vi "LED 7segment Example 1.vi"() -> ()   [LabVIEW 2014]
doc: "Light up 7segment LED."
panel:
  out "error out":errorcluster
  in  "error in":errorcluster
  # "+----------+\n|                |\n|                |\n|                |\n+----------+\n|                |\n|                |\n|                |\n+----------+ +"
  # "pin 9"
  # "pin 8"
  # "pin 10"
  # "pin 7"
  # "pin 6"
  # "pin 3"
  # "pin 4"
  # "pin 2"
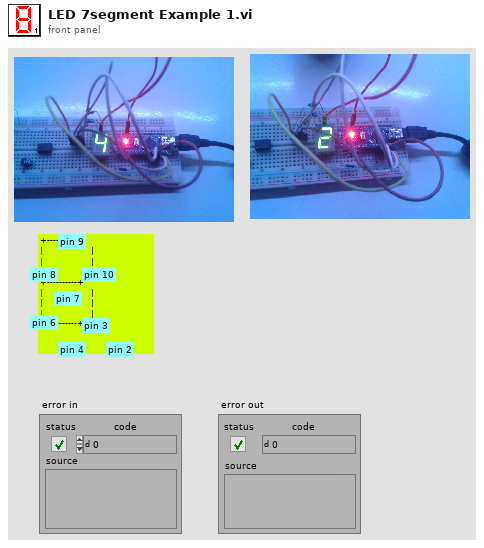
[diagram p1: front panel]
types:
  T1 = enum16{"nothing", "0", "1", "2", "3", "4", "5", "6", "7", "8", "9", "A", "B", "C", "D", "E", "F", "J", "L", "O", "P", "S", "U"}
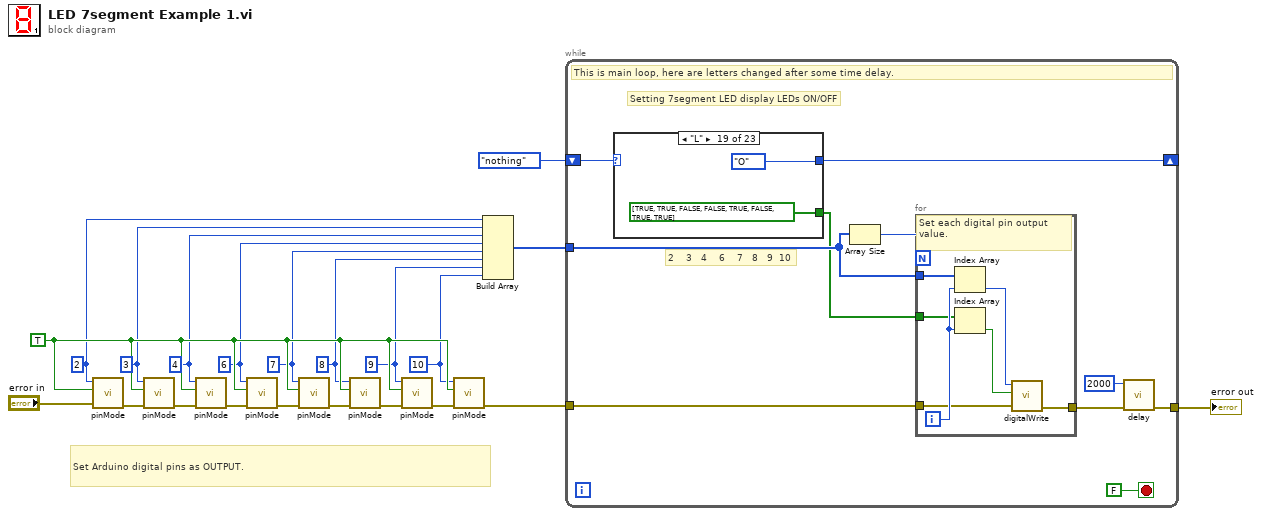
[diagram p0: block diagram]
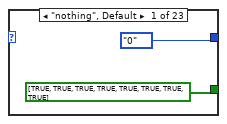
[diagram p2: hidden frame]
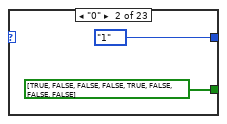
[diagram p3: hidden frame]
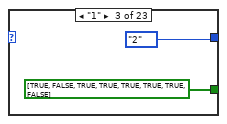
[diagram p4: hidden frame]
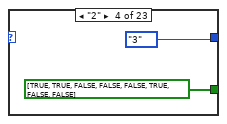
[diagram p5: hidden frame]
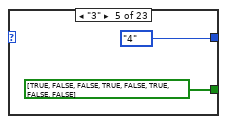
[diagram p6: hidden frame]
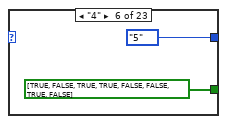
[diagram p7: hidden frame]
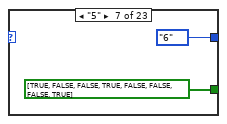
[diagram p8: hidden frame]
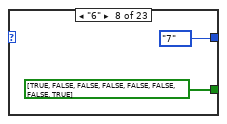
[diagram p9: hidden frame]
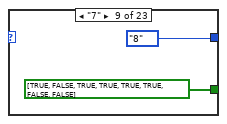
[diagram p10: hidden frame]
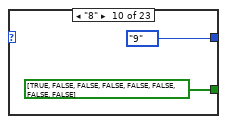
[diagram p11: hidden frame]
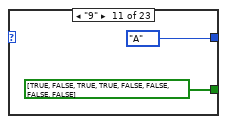
[diagram p12: hidden frame]
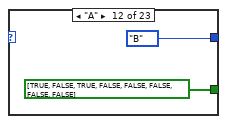
[diagram p13: hidden frame]
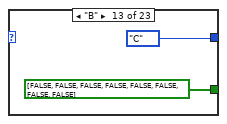
[diagram p14: hidden frame]
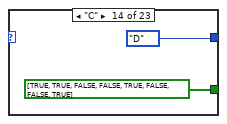
[diagram p15: hidden frame]
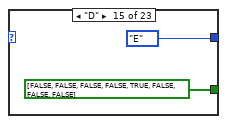
[diagram p16: hidden frame]
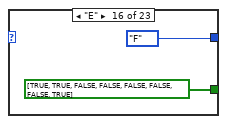
[diagram p17: hidden frame]
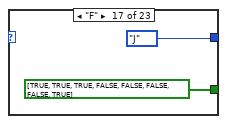
[diagram p18: hidden frame]
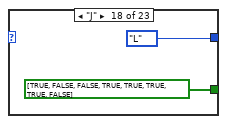
[diagram p19: hidden frame]
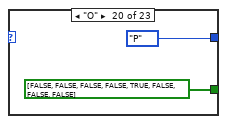
[diagram p20: hidden frame]
diagram:
  w3 = 10 ("pin number")
  w4 = 9 ("pin number")
  w5 = 8 ("pin number")
  w6 = 7 ("pin number")
  w7 = 6 ("pin number")
  w8 = 4 ("pin number")
  w9 = 3 ("pin number")
  w10 = 2 ("pin number")
  w13 = TRUE ("output?")
  # "Set Arduino digital pins as OUTPUT."
  n1 = call <vilib>:"pinMode.vi"("Error In"="error in", "output?"=w13, "pin number"=w10) -> ("Error Out"=w20:errorcluster)  [unwired: 8 in]
  n2 = call <vilib>:"pinMode.vi"("Error In"=w20, "output?"=w13, "pin number"=w9) -> ("Error Out"=w14:errorcluster)  [unwired: 8 in]
  n3 = call <vilib>:"pinMode.vi"("Error In"=w14, "output?"=w13, "pin number"=w8) -> ("Error Out"=w19:errorcluster)  [unwired: 8 in]
  n4 = call <vilib>:"pinMode.vi"("Error In"=w19, "output?"=w13, "pin number"=w7) -> ("Error Out"=w18:errorcluster)  [unwired: 8 in]
  n5 = call <vilib>:"pinMode.vi"("Error In"=w18, "output?"=w13, "pin number"=w6) -> ("Error Out"=w16:errorcluster)  [unwired: 8 in]
  n6 = call <vilib>:"pinMode.vi"("Error In"=w16, "output?"=w13, "pin number"=w5) -> ("Error Out"=w15:errorcluster)  [unwired: 8 in]
  n7 = call <vilib>:"pinMode.vi"("Error In"=w15, "output?"=w13, "pin number"=w4) -> ("Error Out"=w17:errorcluster)  [unwired: 8 in]
  n8 = call <vilib>:"pinMode.vi"("Error In"=w17, "output?"=w13, "pin number"=w3) -> ("Error Out"=w11:errorcluster)  [unwired: 8 in]
  n9 = Build Array(w10, w9, w8, w7, w6, w5, w4, w3) -> (w2:i32[])
  n10 = while {
    tunnel: [w30] -> w21
    tunnel: w11 -> [w27]
    tunnel: w2 -> [w28]
    shift-right: [w23] -> _
    shift-left: T1."nothing" -> [w24]
    stop <- FALSE stop-if-true
    # "Setting 7segment LED display LEDs ON/OFF"
    # "2    3   4    6    7   8   9  10"
    # "This is main loop, here are letters changed after some time delay."
    n11 = case shown="\"L\"" w24 {
      tunnel: [T1."0" T1."1" T1."2" T1."3" T1."4" T1."5" T1."6" T1."7" T1."8" T1."9" T1."A" T1."B" T1."C" T1."D" T1."E" T1."F" T1."J" T1."L" T1."O" T1."P" T1."S" T1."U" T1."nothing"] -> w23
      tunnel: [bool[] [TRUE, TRUE, TRUE, TRUE, TRUE, TRUE, TRUE, TRUE] bool[] [TRUE, FALSE, FALSE, FALSE, TRUE, FALSE, FALSE, FALSE] bool[] [TRUE, FALSE, TRUE, TRUE, TRUE, TRUE, TRUE, FALSE] bool[] [TRUE, TRUE, FALSE, FALSE, FALSE, TRUE, FALSE, FALSE] bool[] [TRUE, FALSE, FALSE, TRUE, FALSE, TRUE, FALSE, FALSE] bool[] [TRUE, FALSE, TRUE, TRUE, FALSE, FALSE, TRUE, FALSE] bool[] [TRUE, FALSE, FALSE, TRUE, FALSE, FALSE, FALSE, TRUE] bool[] [TRUE, FALSE, FALSE, FALSE, FALSE, FALSE, FALSE, TRUE] bool[] [TRUE, FALSE, TRUE, TRUE, TRUE, TRUE, FALSE, FALSE] bool[] [TRUE, FALSE, FALSE, FALSE, FALSE, FALSE, FALSE, FALSE] bool[] [TRUE, FALSE, TRUE, TRUE, FALSE, FALSE, FALSE, FALSE] bool[] [TRUE, FALSE, TRUE, FALSE, FALSE, FALSE, FALSE, FALSE] bool[] [FALSE, FALSE, FALSE, FALSE, FALSE, FALSE, FALSE, FALSE] bool[] [TRUE, TRUE, FALSE, FALSE, TRUE, FALSE, FALSE, TRUE] bool[] [FALSE, FALSE, FALSE, FALSE, TRUE, FALSE, FALSE, FALSE] bool[] [TRUE, TRUE, FALSE, FALSE, FALSE, FALSE, FALSE, TRUE] bool[] [TRUE, TRUE, TRUE, FALSE, FALSE, FALSE, FALSE, TRUE] bool[] [TRUE, FALSE, FALSE, TRUE, TRUE, TRUE, TRUE, FALSE] bool[] [TRUE, TRUE, FALSE, FALSE, TRUE, FALSE, TRUE, TRUE] bool[] [FALSE, FALSE, FALSE, FALSE, TRUE, FALSE, FALSE, FALSE] bool[] [TRUE, TRUE, TRUE, FALSE, FALSE, FALSE, FALSE, FALSE] bool[] [TRUE, FALSE, FALSE, TRUE, FALSE, FALSE, FALSE, TRUE] bool[] [TRUE, FALSE, FALSE, FALSE, TRUE, FALSE, TRUE, FALSE]] -> w25
      frame "nothing", Default {
      }
      frame "0" {
      }
      frame "1" {
      }
      frame "2" {
      }
      frame "3" {
      }
      frame "4" {
      }
      frame "5" {
      }
      frame "6" {
      }
      frame "7" {
      }
      frame "8" {
      }
      frame "9" {
      }
      frame "A" {
      }
      frame "B" {
      }
      frame "C" {
      }
      frame "D" {
      }
      frame "E" {
      }
      frame "F" {
      }
      frame "J" {
      }
      frame "L" {
      }
      frame "O" {
      }
      frame "P" {
      }
      frame "S" {
      }
      frame "U" {
      }
    }
    n12 = Array Size(array=w28) -> (size(s)=w22:i32)
    n13 = for {
      N: w22 -> [_]
      tunnel: w28 -> [w38]
      tunnel: w27 -> [w35]
      tunnel: [w34] -> w26
      tunnel: w25 -> [w33]
      i -> [w36]
      # "Set each digital pin output value."
      n14 = Index Array(array=w38, index=w36) -> (element=w37:i32)
      n15 = Index Array(array=w33, index=w36) -> (element=w32:bool)
      n16 = call <vilib>:"digitalWrite.vi"("Error In"=w35, "value"=w32, "pin number"=w37) -> ("Error Out"=w34:errorcluster)  [unwired: 8 in]
    }
    n17 = call <vilib>:"delay.vi"("Error In"=w26, "time (ms)"=2000) -> ("Error Out"=w30:errorcluster)  [unwired: 9 in]
  }
  "error out" <- w21
